vi "Detector Get Image.vi"(8 "error in (no error)":errorcluster, 10 "Observation":T1={"Priority"=0, "ID"="", "Observer"="", "Obj Name"="", "Obj Type"="", "RA and DEC String"={"RA"="HH:MM:SS.nnn", "DEC"="DEG:arcmin:arcsec.nn"}, "Filter Wheel 1"="", "Filter Wheel 2"="", "Integration Time"=0.0, "Observation Status"=enum."Error", "Offsets"={"RA"=0.0, "DEC"=0.0, "ROT"=0.0}, "Images"=0, "Dither Options"={"Dither"=enum."None", "Dither Radius"=0.0, "Dither Points"=0, "Dither Phase"=0.0}, "Comment 1"="", "Comment 2"=""}, 11 "PRIME Detector in":refnum<class "PRIME Detector.lvclass">) -> (0 "error out":errorcluster, 1 "FITS Detector Settings":T7, 2 "Images":T8[](array[typedef]) {"Detector #" items=["None", "YJ", "HK"]}, 3 "PRIME Detector out":refnum<class "PRIME Detector.lvclass">, 4 "Message Log":string, 6 "Detector Files":T6)   [LabVIEW 2024, in "PRIME Detector.lvclass"]
uses:
  PRIME Detector.lvclass
  C:/Development/Prime-RIMAS/Detector/Detector Class/Detector Class.lvclass
  Detector Image typedef cluster.ctl
  RIMAS Observation Config.ctl
  Detector cluster Files.ctl
  typedefs/CC cluster Observation.ctl
  Observation Queue/CC enum Observation Status.ctl
  Telescope/CC cluster Telescope Offsets.ctl
  typedefs/CC cluster Observation Dither Options.ctl
  typedefs/CC enum Dither Selection.ctl
  Detector Class.lvclass
  PRIME Detector.lvclass/PRIME Detector.ctl
  ed270338-c6d5-43e5-a287-b31ed10c4701.vi
  81b43f0d-8b71-4fcf-9938-3437e86aa932.vi
panel:
  out "Table":string[](array[string])
  # "Make sure that the timeout is set to exceed the maximal exposure time, otherwise the acuisition fails"
  # "sec"
  # "sec"
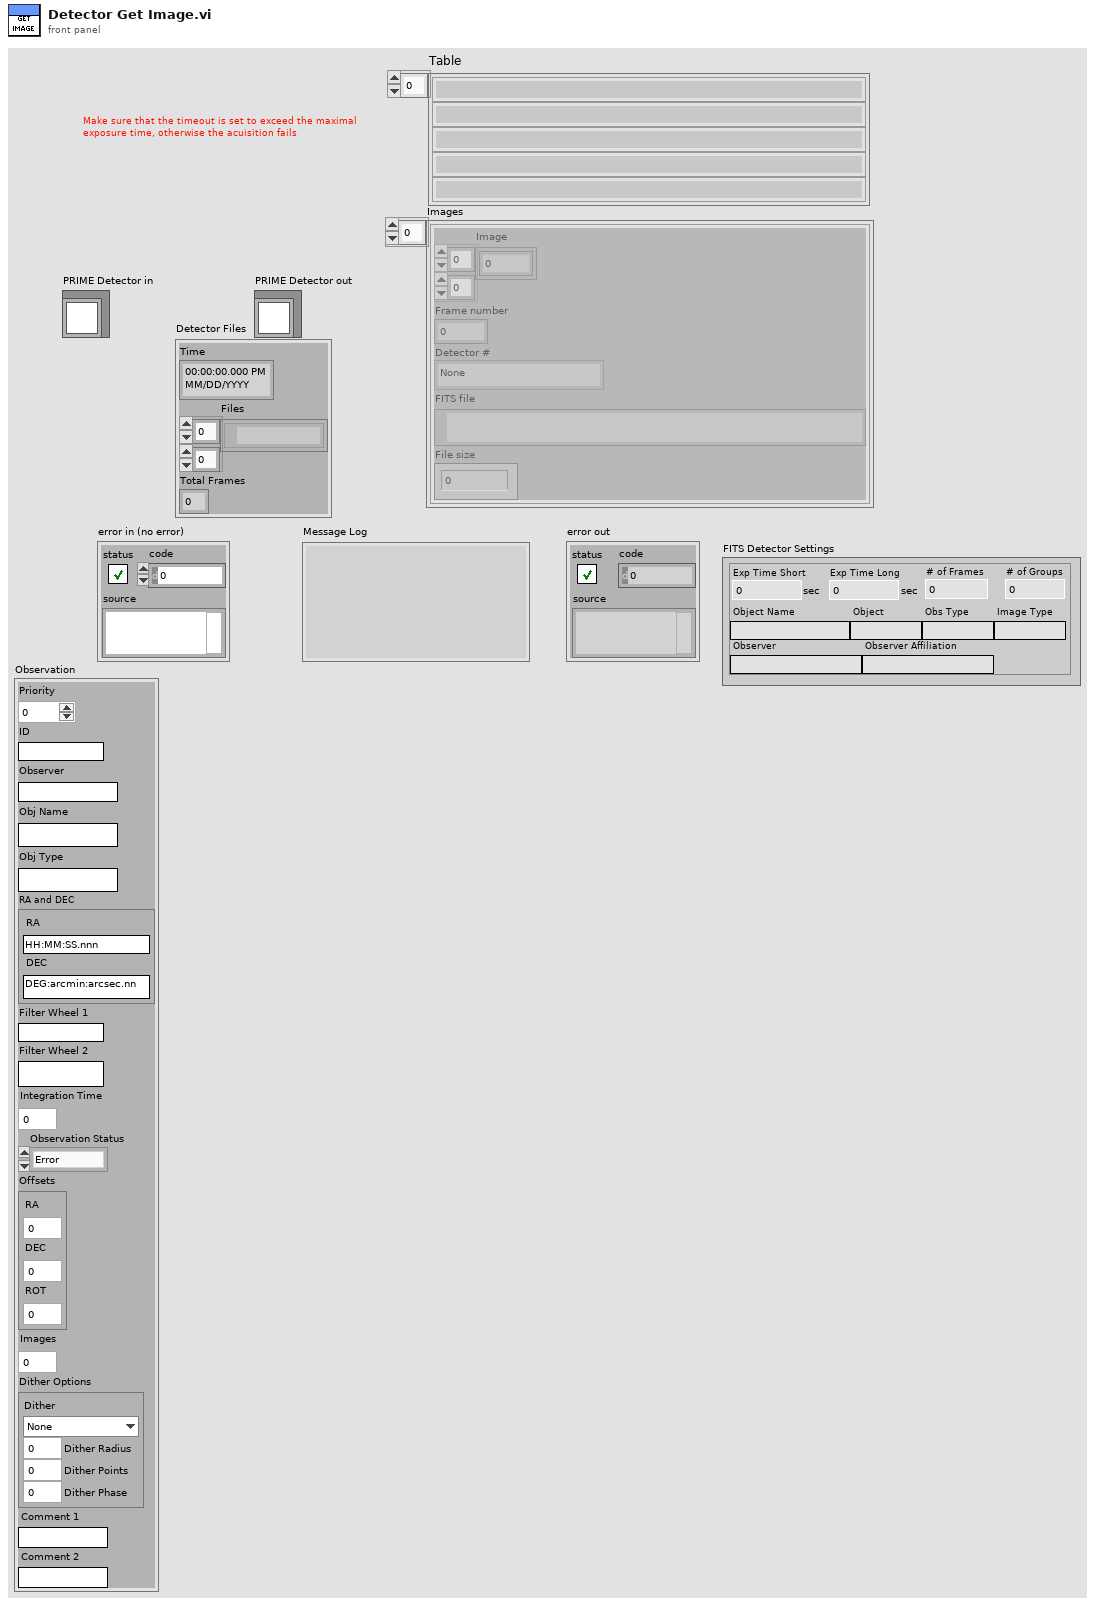
[diagram p1: front panel]
types:
  T1 = typedef "CC cluster Observation.ctl" = cluster{"Priority":i32, "ID":string, "Observer":string, "Obj Name":string, "Obj Type":string, "RA and DEC String":cluster{"RA":string, "DEC":string}, "Filter Wheel 1":string, "Filter Wheel 2":string, "Integration Time":dbl, "Observation Status":T2, "Offsets":T3, "Images":i32, "Dither Options":T4, "Comment 1":string, "Comment 2":string}
  T2 = typedef "CC enum Observation Status.ctl" = enum16{"Ready", "Running", "Done", "Error"}
  T3 = typedef "CC cluster Telescope Offsets.ctl" = cluster{"RA":dbl, "DEC":dbl, "ROT":dbl}
  T4 = typedef "CC cluster Observation Dither Options.ctl" = cluster{"Dither":T5, "Dither Radius":dbl, "Dither Points":i32, "Dither Phase":dbl}
  T5 = typedef "CC enum Dither Selection.ctl" = enum16{"None", "Circle", "Random"}
  T6 = typedef "Detector Class.lvclass/Detector cluster Files.ctl" = cluster{"Time":timestamp, "Files":path[][], "Total Frames":i32}
  T7 = typedef "RIMAS Observation Config.ctl" = cluster{"Exp Time Short":dbl, "# of Frames":dbl, "Exp Time Long":dbl, "# of Groups":dbl, "Object Name":string, "Object":string, "Obs Type":string, "Image Type":string, "Observer":string, "Observer Affiliation":string}
  T8 = typedef "Detector Class.lvclass/Detector Image typedef cluster.ctl" = cluster{"Image":sgl[][], "Frame number":i32, "Detector #":u16, "FITS file":path, "File size":i64}
  T9 = typedef "RIMAS Detector Config.ctl" = cluster{"Detector":u16, "Offsets":u16[][], "Detector Computer":T10, "FITS hdr template0":path, "FITS hdr template1":path, "FITS Data File Path":path, "FITS Detector Settings":T7, "Sim Folder":path, "Integration Mode":T11, "Integration Time":dbl, "Frame Int Time":dbl}
  T10 = typedef "RIMAS Detector Server Config.ctl" = cluster{"Machine":string, "Password":string, "FITS File Path":string, "Port":u16, "Header Path":string, "Name":string}
  T11 = typedef "Detector enum Detector Integration Mode.ctl" = enum16{"SSR", "CDS", "MEAN", "MEDIAN", "MODE", "MIIN", "MAX"}
  T12 = typedef "PRIME Detector cluster Status.ctl" = cluster{"Cmd Start Time":timestamp, "Command":string, "Complete?":bool, "Cmd Complete Time":timestamp, "Exp Time Remaining":dbl, "Total Frames":i32, "Exp Frames":cluster{"CAMERA0":string[], "CAMERA1":string[], "CAMERA2":string[], "CAMERA3":string[]}, "Intermediate Frames":cluster{"CAMERA0":string[], "CAMERA1":string[], "CAMERA2":string[], "CAMERA3":string[]}, "Final Reduced Frame":cluster{"CAMERA0":string, "CAMERA1":string, "CAMERA2":string, "CAMERA3":string}}
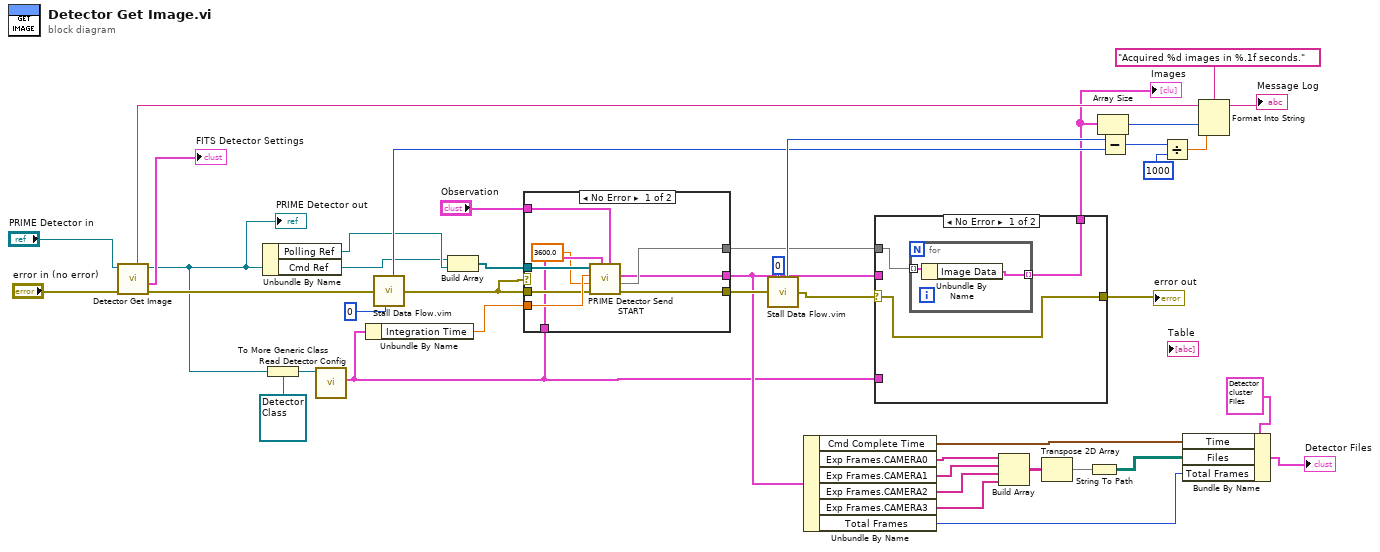
[diagram p0: block diagram]
diagram:
  n1 = call-parent "Detector Get Image.vi"("error in (no error)"="error in (no error)", "Detector Class in"="PRIME Detector in") -> ("error out"=w23:errorcluster, "FITS Detector Settings"=→"FITS Detector Settings":T7, "Detector Class out"=w22:refnum<class "PRIME Detector.lvclass">, "Message Log"=w29:string)  [unwired: 4 in, 2 out]
  "PRIME Detector out" <- w22
  n2 = Unbundle By Name(w22) -> ("Polling Ref"=w25:refnum<k5>, "Cmd Ref"=w17:refnum<k5>)
  n3 = To More Generic Class(target class=refnum<class "Detector Class.lvclass"> refnum ("Detector Class.lvclass"), reference=w22) -> (generic class reference=w39:refnum<class "Detector Class.lvclass">)
  n4 = call-dynamic "Read Detector Config.vi"("Detector Class in"=w39) -> ("Detector Config"=w2:T9)  [unwired: 8 in, 2 out]
  n5 = Unbundle By Name(w2) -> ("Integration Time"=w26:dbl)
  n6 = call "Stall Data Flow.vim"("value in"=w23, "milliseconds to wait"=u32 0) -> ("millisecond timer value"=w36:u32, "value out"=w16:errorcluster)
  n7 = Build Array(w17, w25) -> (w24:refnum<k5>[])
  n8 = case shown="No Error" w16 {
    tunnel: w26 -> [w51 _]
    tunnel: [w46 _] -> w10
    tunnel: w16 -> [w50 w52]
    tunnel: w24 -> [w49 _]
    tunnel: [w48 w52] -> w20
    tunnel: [w47 _] -> w3
    tunnel: w2 -> [w45 _]
    tunnel: "Observation" -> [w44 _]
    frame No Error {
      n9 = call "PRIME Detector Send START.vi"("Observation"=w44, "Detector Config"=w45, "error in (no error)"=w50, "timeout (120s)"=3600.0, "Exposure Time"=w51, "connection ID"=w49) -> ("error out"=w48:errorcluster, "Image Map"=w47:map{string, T8}, "Status out"=w46:T12)  [unwired: 2 in, 1 out]
    }
    frame Error {
    }
  }
  n10 = call "Stall Data Flow.vim"("value in"=w20, "milliseconds to wait"=u32 0) -> ("millisecond timer value"=w37:u32, "value out"=w18:errorcluster)
  n11 = Unbundle By Name(w10) -> ("Cmd Complete Time"=w8:timestamp, "Exp Frames.CAMERA0"=w15:string[], "Exp Frames.CAMERA1"=w14:string[], "Exp Frames.CAMERA2"=w13:string[], "Exp Frames.CAMERA3"=w12:string[], "Total Frames"=w7:i32)
  n12 = case shown="No Error" w18 {
    selector: w18 -> [w53 w58]
    tunnel: w2 -> [_ _]
    tunnel: [w54 _] -> w27
    tunnel: w10 -> [_ _]
    tunnel: [w53 w58] -> w19
    tunnel: w3 -> [w55 _]
    frame No Error {
      n13 = for {
        tunnel: w55 -> [w57] mode=indexing
        tunnel: [w56] -> w54 mode=indexing
        n14 = Unbundle By Name(w57) -> ("Image Data"=w56:T8)
      }
    }
    frame Error {
    }
  }
  "error out" <- w19
  "Images" <- w27
  n15 = Build Array(w15, w14, w13, w12) -> (w11:string[][])
  n16 = Transpose 2D Array(2D array=w11) -> (transposed array=w6:string[][])
  n17 = String To Path(string=w6) -> (path=w5:path[][])
  n18 = Array Size(array=w27) -> (size(s)=w34:i32)
  n19 = Subtract(x=w37, y=w36) -> (x-y=w33:u32)
  n20 = Divide(x=w33, y=u32 1000) -> (x/y=w31:dbl)
  n21 = Bundle By Name(cluster=T6 {"Time"=timestamp(0 s since 1904-01-01), "Files"=[], "Total Frames"=0} ("Detector Files"), "Time"=w8, "Files"=w5, "Total Frames"=w7) -> (→"Detector Files":T6)
  n22 = Format Into String(format string="Acquired %d images in %.1f seconds.", initial string=w29, w34, w31) -> (resulting string=→"Message Log":string)  [unwired: 1 in, 1 out]
